vi "hpanel_generate_user_events.vi"(8 "error in (no error)":errorcluster, 11 "hydraharp_panel in":refnum<class "hydraharp_panel.lvclass">) -> (0 "error out":errorcluster, 2 "events":T1, 3 "hydraharp_panel out":refnum<class "hydraharp_panel.lvclass">)   [LabVIEW 2015, in "hydraharp_panel.lvclass"]
uses:
  hydraharp_panel.lvclass
  hpanel_user_events.ctl
  hpanel_messages_to_panel_from_actor_loop.ctl
  hydraharp_panel.lvclass/hydraharp_panel.ctl
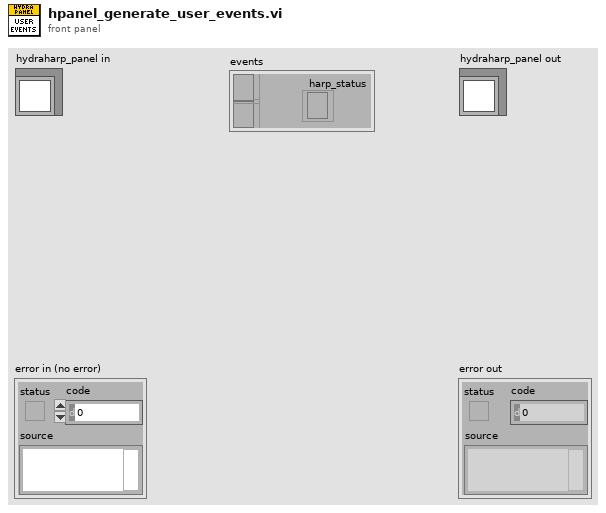
[diagram p1: front panel]
types:
  T1 = typedef "hpanel_user_events.ctl" = cluster{"message_panel":refnum<event-registration>, "stop_fifo_stream":refnum<event-registration>, "harp_status":refnum<event-registration>}
  T2 = typedef "hpanel_messages_to_panel_from_actor_loop.ctl" = enum16{"reenable_tasks"}
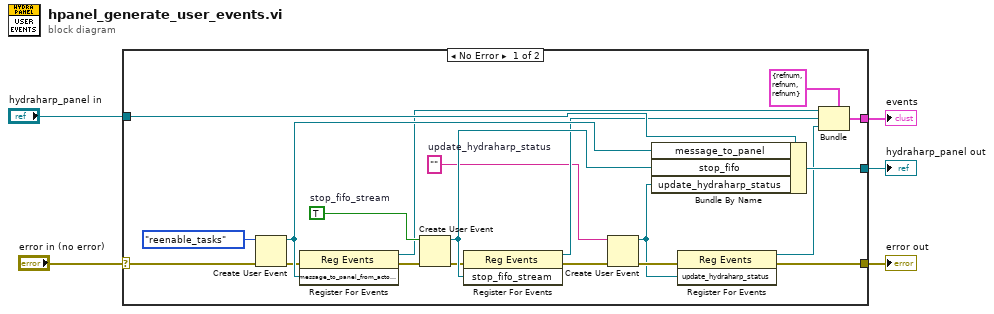
[diagram p0: block diagram]
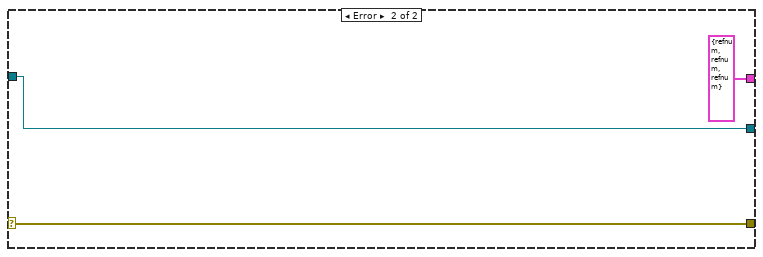
[diagram p2: hidden frame]
diagram:
  n1 = case shown="No Error" "error in (no error)" {
    selector: "error in (no error)" -> [w24 w28]
    tunnel: [w8 w28] -> w4
    tunnel: [w21 w27] -> w2
    tunnel: "hydraharp_panel in" -> [w23 w27]
    tunnel: [w15 T1 {"message_panel"=refnum, "stop_fifo_stream"=refnum, "harp_status"=refnum} ("output cluster")] -> w1
    frame No Error {
      w10 = ""  # update_hydraharp_status
      w20 = TRUE  # stop_fifo_stream
      n2 = Create User Event(user event datatype=hpanel_messages_to_panel_from_actor_loop."reenable_tasks" ("message_to_panel_from_actor_loop"), error in=w24) -> (user event=w22:refnum<user-event>, error out=w14:errorcluster)
      n3 = register-events(error in=w14, w22) -> (reference out=w17:refnum<event-registration>, error out=w13:errorcluster)  [unwired: 1 in]
      n4 = Create User Event(user event datatype=w20, error in=w13) -> (user event=w19:refnum<user-event>, error out=w12:errorcluster)
      n5 = register-events(error in=w12, w19) -> (reference out=w18:refnum<event-registration>, error out=w11:errorcluster)  [unwired: 1 in]
      n6 = Create User Event(user event datatype=w10, error in=w11) -> (user event=w7:refnum<user-event>, error out=w9:errorcluster)
      n7 = Bundle By Name(cluster=w23, "message_to_panel"=w22, "stop_fifo"=w19, "update_hydraharp_status"=w7) -> (w21:refnum<class "hydraharp_panel.lvclass">)
      n8 = register-events(error in=w9, w7) -> (reference out=w6:refnum<event-registration>, error out=w8:errorcluster)  [unwired: 1 in]
      n9 = Bundle(cluster=T1 {"message_panel"=refnum, "stop_fifo_stream"=refnum, "harp_status"=refnum} ("output cluster"), "message_panel"=w17, "stop_fifo_stream"=w18, "harp_status"=w6) -> (w15:T1)
    }
    frame Error {
    }
  }
  "error out" <- w4
  "hydraharp_panel out" <- w2
  "events" <- w1
